vi "Update Channels.vi"(8 "error in":errorcluster, 10 "Channels to Create":T2[](array[typedef]), 11 "VI Map":T1) -> (0 "error out":errorcluster)   [LabVIEW 2021, in "Plugin Generator.lvlib"]
uses:
  Channels/ChannelRegistrar/typedef/Channel Definition.ctl
  <vilib>/CIF Foundation/CIF Channels Core/CIFChannels/Typedef/Direction.ctl
  Channels/ChannelRegistrar/typedef/Registered Channel Types.ctl
  <vilib>/Utility/traverseref.llb/TRef TravTarget.ctl
  Plugin Generator.lvlib
  <vilib>/Utility/traverseref.llb/VI Scripting - Traverse.lvlib
  Channels/ChannelRegistrar/ChannelRegistrar.lvlib
  <vilib>/CIF Foundation/CIF Channels Core/CIFChannels/CIFChannels.lvclass
  <vilib>/CIF Foundation/CIF LabVIEW Scripting/Update Enum/Update Enum.lvlib
  <vilib>/CIF Foundation/CIF LabVIEW Scripting/LV Scripting/LV Scripting Utilities.lvlib
  <vilib>/CIF Foundation/CIF LabVIEW Scripting/LV Scripting/Typedef/Errors.ctl
  Channels/ChannelRegistrar/typedef/Channel Definition for Scripting.ctl
  <vilib>/CIF Foundation/CIF LabVIEW Scripting/LV Scripting/Typedef/VI Map.ctl
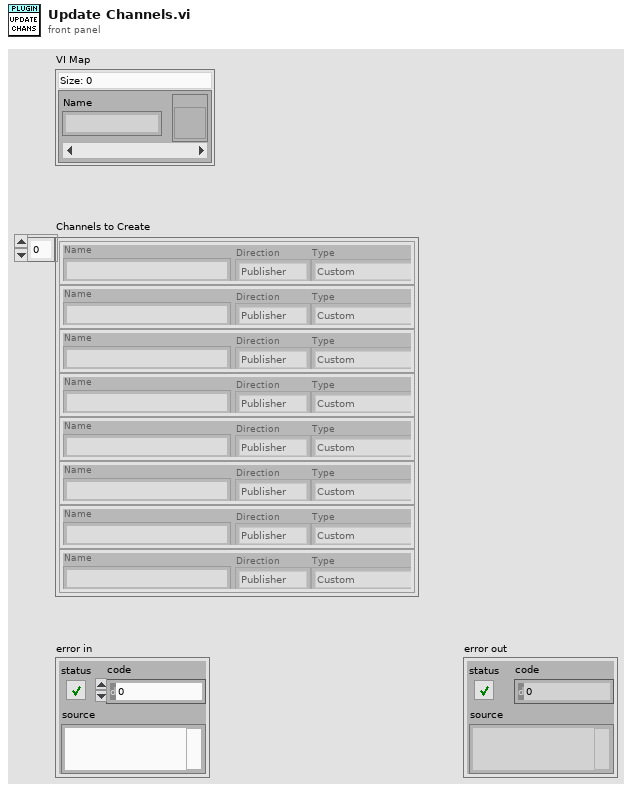
[diagram p1: front panel]
types:
  T1 = typedef "LV Scripting Utilities.lvlib/VI Map.ctl" = map{string, refnum<vi>}
  T2 = typedef "ChannelRegistrar.lvlib/Channel Definition for Scripting.ctl" = cluster{"Name":string, "Direction":T3, "Type":T4}
  T3 = typedef "CIFChannels.lvclass/Direction.ctl" = enum16{"Publisher", "Subscriber"}
  T4 = typedef "ChannelRegistrar.lvlib/Registered Channel Types.ctl" = enum16{"Custom", "Double_Tag", "I64_Tag", "U64_Tag", "U8_FIFO", "CAN_FIFO", "L2Enet_FIFO", "DAQ_FIFO", "Universal_FIFO", "String_Tag"}
  T5 = typedef "ChannelRegistrar.lvlib/Channel Definition.ctl" = cluster{"Name":string, "Direction":T3, "Type":T4, "Custom Config Data":u8[]}
  T6 = typedef "TRef TravTarget.ctl" = enum16{"FP", "BD", "Other"}
  T7 = typedef "Errors.ctl" = enum16{"Missing Version Changes", "Item not found"}
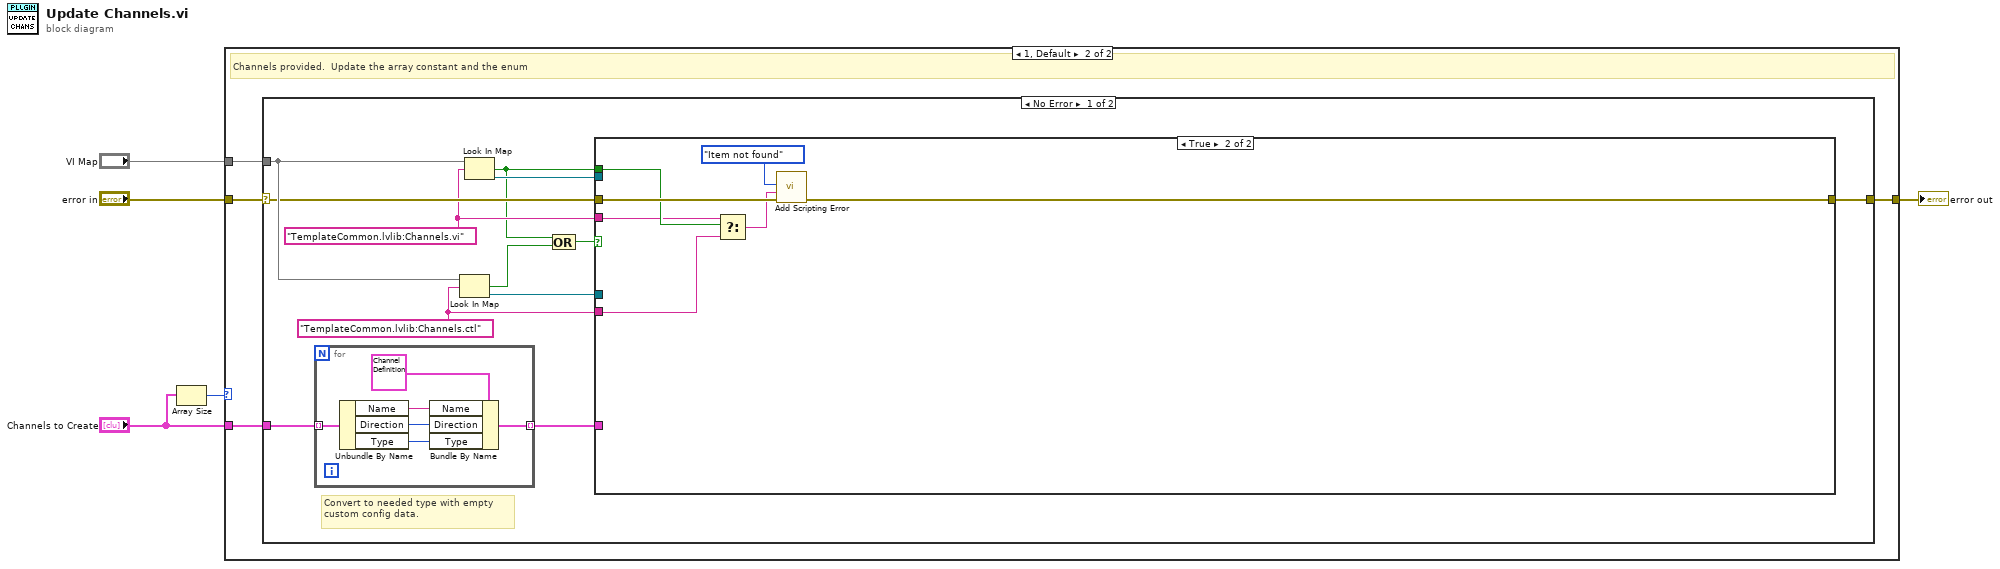
[diagram p0: block diagram]
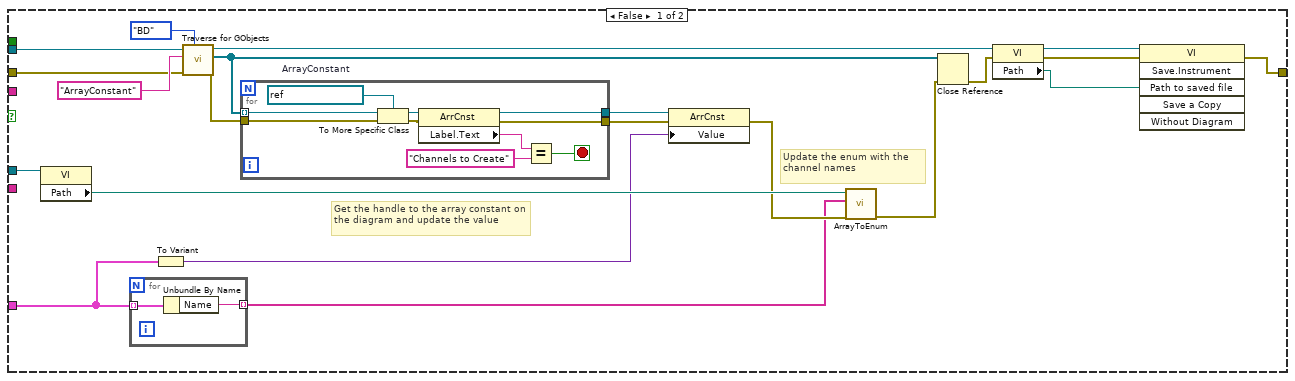
[diagram p3: hidden frame]
diagram:
  n1 = Array Size(array="Channels to Create") -> (size(s)=w1:i32)
  n2 = case shown="1, Default" w1 {
    tunnel: "VI Map" -> [_ w10]
    tunnel: "error in" -> [w6 w9]
    tunnel: [w6 w8] -> w3
    tunnel: "Channels to Create" -> [_ w7]
    frame 0 {
      # "No channel list provided. Skip scripting"
    }
    frame 1, Default {
      # "Channels provided.  Update the array constant and the enum"
      n3 = case shown="No Error" w9 {
        selector: w9 -> [w14 w69]
        tunnel: [w22 w69] -> w8
        tunnel: w10 -> [w20 _]
        tunnel: w7 -> [w16 _]
        frame No Error {
          w12 = "TemplateCommon.lvlib:Channels.ctl" ("String")
          w13 = "TemplateCommon.lvlib:Channels.vi" ("String")
          # "Convert to needed type with empty custom config data."
          n4 = for {
            tunnel: w16 -> [w28] mode=indexing
            tunnel: [w23] -> w15 mode=indexing
            n5 = Unbundle By Name(w28) -> ("Name"=w26:string, "Direction"=w25:T3, "Type"=w24:T4)
            n6 = Bundle By Name(cluster=T5 {"Name"="testme", "Direction"=enum."Subscriber", "Type"=enum."L2Enet_FIFO", "Custom Config Data"=[]} ("Channel Definition"), "Name"=w26, "Direction"=w25, "Type"=w24) -> (w23:T5)
          }
          n7 = Look In Map(map=w20, key=w12) -> (key not found?=w19:bool, value=w17:refnum<vi>)  [unwired: 1 in]
          n8 = Look In Map(map=w20, key=w13) -> (key not found?=w11:bool, value=w21:refnum<vi>)  [unwired: 1 in]
          n9 = Compound Arithmetic op=OR(w11, w19) -> (w18:bool)
          n10 = case shown="True" w18 {
            tunnel: [w41 w66] -> w22
            tunnel: w21 -> [w40 _]
            tunnel: w14 -> [w39 w67]
            tunnel: w17 -> [w35 _]
            tunnel: w15 -> [w30 _]
            tunnel: w13 -> [_ w64]
            tunnel: w12 -> [_ w63]
            tunnel: w11 -> [_ w65]
            frame False {
              # "Update the enum with the channel names"
              # "Get the handle to the array constant on the diagram and update the value"
              n11 = property class="VI"(reference=w35) -> ("Path"=w34:path)  [unwired: 1 in, 2 out]
              n12 = for {
                tunnel: w30 -> [w51] mode=indexing
                tunnel: [w50] -> w29 mode=indexing
                n13 = Unbundle By Name(w51) -> ("Name"=w50:string)
              }
              n14 = To Variant(anything=w30) -> (Variant=w31:variant)
              n15 = call <vilib>:"Traverse for GObjects.vi"("Traverse Target"=TRef_TravTarget."BD", "error in (no error)"=w39, "Class Name"="ArrayConstant", "VI Refnum"=w40) -> ("error out"=w38:errorcluster, "References"=w47:refnum<vi>[], "dup VI Refnum"=w44:refnum<vi>)  [unwired: 4 in, 1 out]
              n16 = for {
                tunnel: w47 -> [w61] mode=indexing
                tunnel: [w58] -> w37
                tunnel: [w57] -> w36
                tunnel: w38 -> [w56]
                stop <- w52 stop-if-true
                w60 = refnum<vi> refnum  # ArrayConstant
                n17 = To More Specific Class(target class=w60, reference=w61, error in=w56) -> (specific class reference=w59:refnum<vi>, error out=w55:errorcluster)
                n18 = property class="ArrCnst"(reference=w59, error in=w55) -> (reference out=w58:refnum<vi>, error out=w57:errorcluster, "Label.Text"=w54:string)
                n19 = Equal?(x=w54, y="Channels to Create") -> (x = y?=w52:bool)
              }
              n20 = property class="ArrCnst"(reference=w37, error in=w36, "Value"=w31) -> (error out=w33:errorcluster)  [unwired: 1 out]
              n21 = call <vilib>:"ArrayToEnum.vi"("Error In"=w33, "Enum Strings"=w29, "Enum Path"=w34) -> ("Error Out"=w32:errorcluster)  [unwired: 8 in]
              n22 = Close Reference(reference=w47, error in (no error)=w32) -> (error out=w43:errorcluster)
              n23 = property class="VI"(reference=w44, error in=w43) -> (reference out=w49:refnum<vi>, error out=w48:errorcluster, "Path"=w42:path)
              n24 = invoke class="VI" method="Save.Instrument"(reference=w49, error in=w48, "Path to saved file"=w42) -> (error out=w41:errorcluster)  [unwired: 3 in, 5 out]
            }
            frame True {
              n25 = Select(t=w64, s=w65, f=w63) -> (s? t:f=w62:string)
              n26 = call <vilib>:"Add Scripting Error.vi"("error in (no error)"=w67, "String to Append"=w62, "Error"=Errors."Item not found") -> ("error out"=w66:errorcluster)  [unwired: 8 in]
            }
          }
        }
        frame Error {
        }
      }
    }
  }
  "error out" <- w3
